vi "countrate.vi"() -> ()   [LabVIEW 2015]
uses:
  <vilib>/Platform/TimedLoop/XDataNode/timing_clust.ctl
  <vilib>/Platform/TimedLoop/XDataNode/nitl_modes.ctl
  <vilib>/Platform/TimedLoop/XDataNode/wakeup.ctl
  <vilib>/Utility/file.llb/Write Delimited Spreadsheet (I64).vi
  <vilib>/platform/TimedLoop/XDataNode/XDataNode.xnode
  <vilib>/Platform/TimedLoop/XDataNode/XDNodeRunTimeDep.lvlib
panel:
  in  "File to Save":path
  out "Waveform Graph":i32[](graph)
  in  "Total Time [s]":i32
  in  "Period [s]":i64
  in  "stop":bool
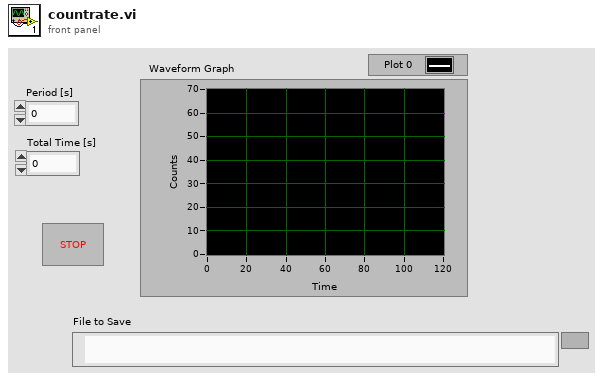
[diagram p1: front panel]
types:
  T1 = typedef "XDNodeRunTimeDep.lvlib/timing_clust.ctl" = cluster{"Expected End [f-1]":u64, "Actual End [f-1]":u64, "Finished Late? [f-1]":bool, "Expected End [i-1]":u64, "Actual End [i-1]":u64, "Finished Late? [i-1]":bool, "Expected Start [i]":u64, "Actual Start [i]":u64, "Expected Start [f]":u64, "Actual Start [f]":u64, "Source Name":string, "Structure Name":string, "Period":i64, "Deadline":i64, "Offset":i64, "Start":i64, "Priority":i32, "Timeout":i32, "Mode":T2, "Wakeup Reason":T3, "Error":errorcluster, "Source Type":string, "Secondary Source Type":string, "Global End Time":u64, "Global Start Time":u64, "Frame Duration":u64, "Iteration Duration":u64, "Assigned CPU":i32, "I/O Scan Engine Mode":u32}
  T2 = typedef "XDNodeRunTimeDep.lvlib/nitl_modes.ctl" = enum32{"No Change", "Process missed periods, maintain original phase", "Discard missed periods, maintain original phase", "Process missed periods, ignore original phase", "Discard missed periods, ignore original phase"}
  T3 = typedef "XDNodeRunTimeDep.lvlib/wakeup.ctl" = enum32{"Normal", "Aborted", "Asynchronous wakeup", "Timing source error", "Timed loop error", "Timeout"}
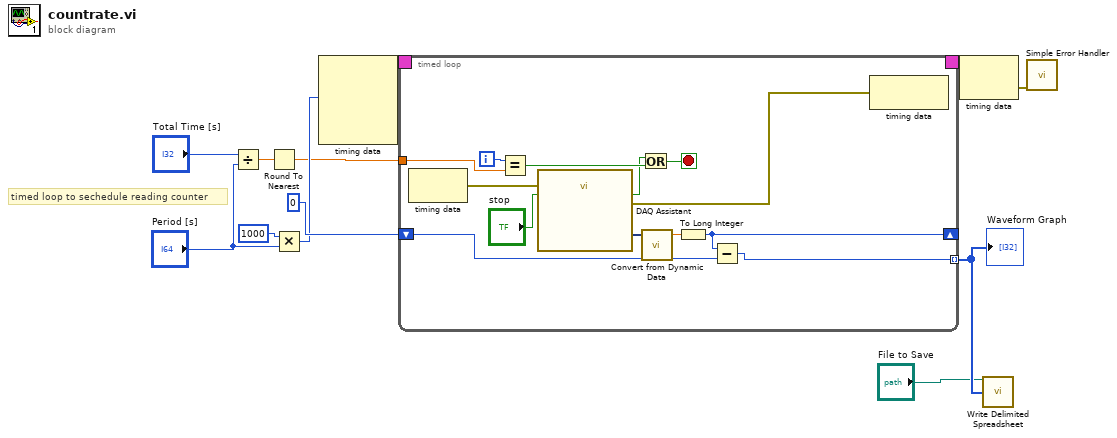
[diagram p0: block diagram]
diagram:
  # "timed loop to sechedule reading counter"
  n1 = Divide(x="Total Time [s]", y="Period [s]") -> (x/y=w2:dbl)
  n2 = Round To Nearest(number=w2) -> (nearest integer value=w1:dbl)
  n3 = Multiply(x=i64 1000, y="Period [s]") -> (x*y=w8:i64)
  n4 = node-c288(w8) -> (w12:T1)  [unwired: 3 in]
  n5 = timed-loop {
    timing: w12 -> [_]
    timing-out: [_] -> w11
    shift-right: [w22] -> _
    shift-left: 0 -> [w24]
    tunnel: [w14] -> w6 mode=indexing
    tunnel: w1 -> [w13]
    i -> [w18]
    stop <- w17 stop-if-true
    n6 = node-c288() -> (w19:errorcluster)  [unwired: 1 in]
    n7 = Equal?(x=w18, y=w13) -> (x = y?=w16:bool)
    n8 = call "DAQ Assistant"("error in"=w19, "stop (F)"="stop") -> ("data"=w25:dynamicdata, "stopped"=w15:bool, "error out"=w20:errorcluster)  [unwired: 14 in, 1 out]
    n9 = Or(x=w15, y=w16) -> (x .or. y?=w17:bool)
    n10 = call "Convert from Dynamic Data"("Dynamic Data Type"=w25) -> ("Scalar"=w21:dbl)  [unwired: 3 in]
    n11 = To Long Integer(number=w21) -> (32bit integer=w22:i32)
    n12 = Subtract(x=w22, y=w24) -> (x-y=w14:i32)
    n13 = node-c288(w20) -> ()  [unwired: 1 out]
  }
  "Waveform Graph" <- w6
  n14 = node-c288(w11) -> (w9:errorcluster)
  n15 = call-poly <vilib>:"Write Delimited Spreadsheet.vi"("file path (dialog if empty)"="File to Save", "1D data"=w6) -> ()  [unwired: 12 in, 2 out]
  n16 = call <vilib>:"Simple Error Handler.vi"("error in (no error)"=w9) -> ()  [unwired: 4 in, 5 out]
